vi "detTSetpointFromProfile.vi"(8 "error in (no error)":errorcluster, 11 "TestMonitor in":refnum<class "TestMonitor.lvclass">) -> (0 "error out":errorcluster, 2 "temperatureSetpoint":dbl[unit]=273.15, 3 "TestMonitor out":refnum<class "TestMonitor.lvclass">)   [LabVIEW 2013, in "TestMonitor.lvclass"]
uses:
  TestMonitor.lvclass
  TestMonitor.lvclass/TestMonitor.ctl
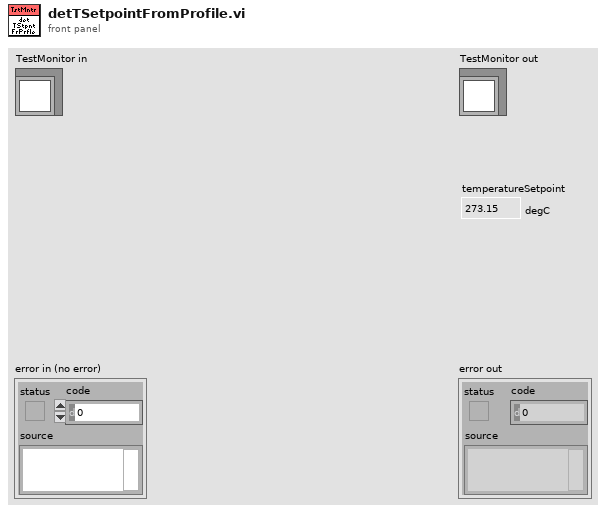
[diagram p1: front panel]
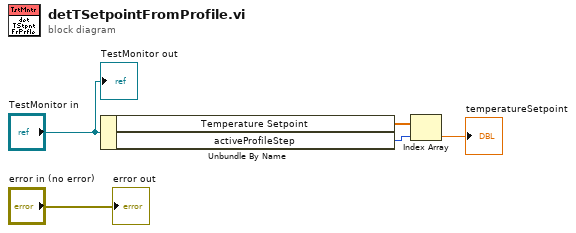
[diagram p0: block diagram]
diagram:
  n1 = Unbundle By Name("TestMonitor in") -> ("Temperature Setpoint"=w3:dbl[unit][], "activeProfileStep"=w2:u32)
  n2 = Index Array(array=w3, index=w2) -> (element=→"temperatureSetpoint":dbl[unit])
  "error out" <- "error in (no error)"
  "TestMonitor out" <- "TestMonitor in"
